vi "CompareInitConfig(PortSpeed).vi"(10 "PortSpeed - existing":u32[](array[ring]) items=["FDX_100MBIT"=0, "FDX_10MBIT"=1, "FDX_AUTO_100MBIT"=2, "FDX_AUTO_10MBIT"=3, "FDX_1000MBIT"=5], 11 "PortSpeed - new":T1 {"Port4SpeedIn" items=["FDX_100MBIT"=0, "FDX_10MBIT"=1, "FDX_AUTO_100MBIT"=2, "FDX_AUTO_10MBIT"=3, "FDX_1000MBIT"=5]; "Port3SpeedIn" items=["FDX_100MBIT"=0, "FDX_10MBIT"=1, "FDX_AUTO_100MBIT"=2, "FDX_AUTO_10MBIT"=3, "FDX_1000MBIT"=5]; "Port2SpeedIn" items=["FDX_100MBIT"=0, "FDX_10MBIT"=1, "FDX_AUTO_100MBIT"=2, "FDX_AUTO_10MBIT"=3, "FDX_1000MBIT"=5]; "Port1SpeedIn" items=["FDX_100MBIT"=0, "FDX_10MBIT"=1, "FDX_AUTO_100MBIT"=2, "FDX_AUTO_10MBIT"=3, "FDX_1000MBIT"=5]}) -> (2 "not equal":bool, 3 "PortSpeed - new out":T1 {"Port4SpeedIn" items=["FDX_100MBIT"=0, "FDX_10MBIT"=1, "FDX_AUTO_100MBIT"=2, "FDX_AUTO_10MBIT"=3, "FDX_1000MBIT"=5]; "Port3SpeedIn" items=["FDX_100MBIT"=0, "FDX_10MBIT"=1, "FDX_AUTO_100MBIT"=2, "FDX_AUTO_10MBIT"=3, "FDX_1000MBIT"=5]; "Port2SpeedIn" items=["FDX_100MBIT"=0, "FDX_10MBIT"=1, "FDX_AUTO_100MBIT"=2, "FDX_AUTO_10MBIT"=3, "FDX_1000MBIT"=5]; "Port1SpeedIn" items=["FDX_100MBIT"=0, "FDX_10MBIT"=1, "FDX_AUTO_100MBIT"=2, "FDX_AUTO_10MBIT"=3, "FDX_1000MBIT"=5]})   [LabVIEW 2020, in "AIM664LV.lvlib"]
uses:
  AIM664LV.lvlib
  _controls/initialize_PortSpeed.ctl
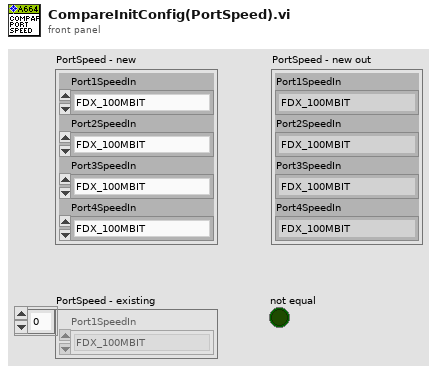
[diagram p1: front panel]
types:
  T1 = typedef "AIM664LV.lvlib/initialize_PortSpeed.ctl" = cluster{"Port1SpeedIn":u32, "Port2SpeedIn":u32, "Port3SpeedIn":u32, "Port4SpeedIn":u32}
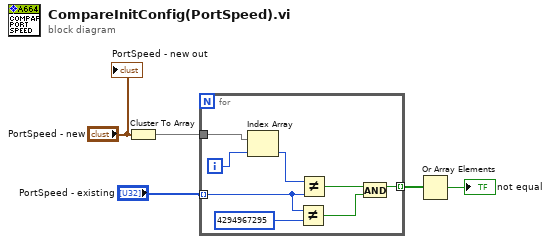
[diagram p0: block diagram]
diagram:
  n1 = Cluster To Array(cluster="PortSpeed - new") -> (array=w3:u32[])
  n2 = for {
    tunnel: "PortSpeed - existing" -> [w9] mode=indexing
    tunnel: w3 -> [w13]
    tunnel: [w7] -> w1 mode=indexing
    i -> [w12]
    n3 = Index Array(array=w13, index=w12) -> (element=w11:u32)
    n4 = Not Equal?(x=w9, y=u32 4294967295) -> (x != y?=w6:bool)
    n5 = Not Equal?(x=w11, y=w9) -> (x != y?=w10:bool)
    n6 = And(x=w10, y=w6) -> (x .and. y?=w7:bool)
  }
  n7 = Or Array Elements(Boolean array=w1) -> (logical OR=→"not equal":bool)
  "PortSpeed - new out" <- "PortSpeed - new"
